vi "Read Test Case object from front panel control.vi"(8 "error in (no error)":errorcluster, 11 "LUnit Test Case In":refnum<class "LUnit Test Case.lvclass">) -> (0 "error out":errorcluster, 3 "LUnit Test Case Out":refnum<class "LUnit Test Case.lvclass">)   [LabVIEW 2020, in "LUnit Test Case.lvclass"]
uses:
  LUnit Test Case.lvclass
  LUnit Test Case.lvclass/LUnit Test Case.ctl
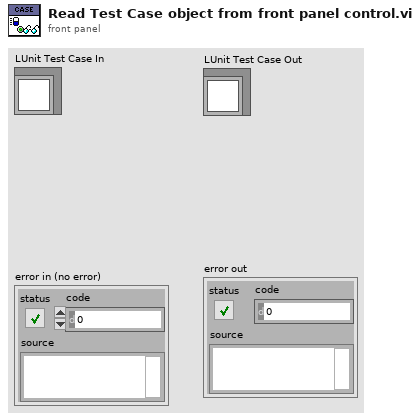
[diagram p1: front panel]
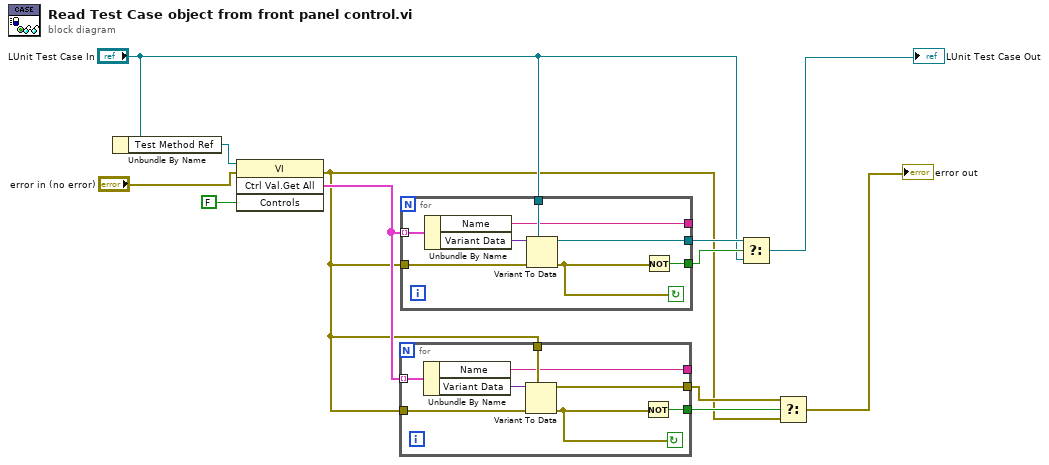
[diagram p0: block diagram]
diagram:
  n1 = Unbundle By Name("LUnit Test Case In") -> ("Test Method Ref"=w6:refnum<vi>)
  n2 = invoke on="Invoke Node" class="VI" method="Ctrl Val.Get All"(reference=w6, error in="error in (no error)", "Controls"=FALSE) -> (error out=w2:errorcluster, "Get All Control Values Variant"=w5:cluster{"Name":string, "Variant Data":variant}[])  [unwired: 1 in, 2 out]
  n3 = for {
    tunnel: w5 -> [w20] mode=indexing
    tunnel: w2 -> [w18]
    tunnel: [w17] -> _
    tunnel: [w13] -> w4
    tunnel: [w15] -> w3
    tunnel: w2 -> [w14]
    stop <- w16 continue-if-true
    n4 = Unbundle By Name(w20) -> ("Name"=w17:string, "Variant Data"=w19:variant)
    n5 = Variant To Data(error in=w14, type=w18, Variant=w19) -> (data=w15:errorcluster, error out=w16:errorcluster)
    n6 = Not(x=w16) -> (.not. x?=w13:bool)
  }
  n7 = for {
    tunnel: w5 -> [w28] mode=indexing
    tunnel: "LUnit Test Case In" -> [w26]
    tunnel: [w25] -> _
    tunnel: [w21] -> w9
    tunnel: [w23] -> w8
    tunnel: w2 -> [w22]
    stop <- w24 continue-if-true
    n8 = Unbundle By Name(w28) -> ("Name"=w25:string, "Variant Data"=w27:variant)
    n9 = Variant To Data(error in=w22, type=w26, Variant=w27) -> (data=w23:refnum<class "LUnit Test Case.lvclass">, error out=w24:errorcluster)
    n10 = Not(x=w24) -> (.not. x?=w21:bool)
  }
  n11 = Select(t=w8, s=w9, f="LUnit Test Case In") -> (s? t:f=→"LUnit Test Case Out":refnum<class "LUnit Test Case.lvclass">)
  n12 = Select(t=w3, s=w4, f=w2) -> (s? t:f=→"error out":errorcluster)
